vi "Status.Builder.State.New.vi"(8 "error in (no error)":errorcluster, 11 "Builder State in":refnum<class "Status.Builder.State.lvclass">) -> (0 "error out":errorcluster, 3 "Builder State out":refnum<class "Status.Builder.State.lvclass">)   [LabVIEW 2016, in "DSF.Engine.lvlib" / "Status.Builder.State.lvclass"]
uses:
  Status.Builder.State.lvclass
  C:/Git/Sourcetree/DSF/Source/Submodules/Memory/Source/Classes/Standard Types/Memory.Pointer.U8.lvclass
  Submodules/Memory/Source/Classes/Internal/Memory.Pointer.Internal.New.vi
  Submodules/Memory/Source/Classes/Internal/Memory.Pointer.Internal.New.1B.vi
  Submodules/Memory/Source/Classes/Standard Types/Memory.Pointer.U8.lvclass
  C:/Git/Sourcetree/DSF/Source/Submodules/Memory/Source/Classes/Internal/Memory.Pointer.Internal.lvclass
  Submodules/Memory/Source/Classes/Internal/Memory.Pointer.Internal.Allocate.vi
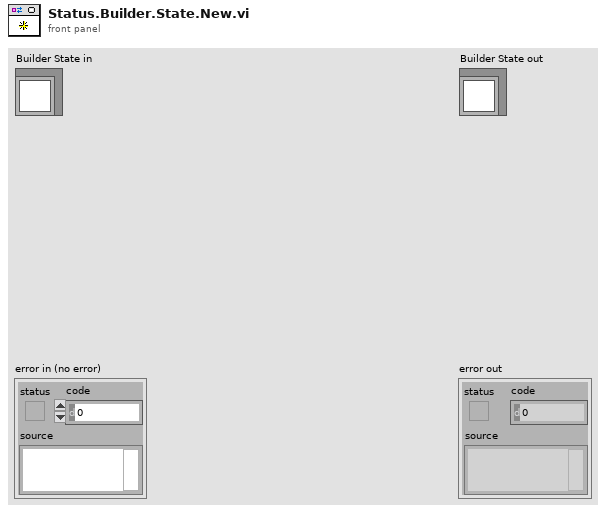
[diagram p1: front panel]
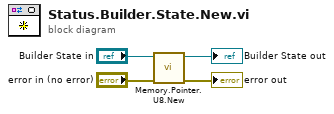
[diagram p0: block diagram]
diagram:
  n1 = call "Memory.Pointer.U8.New.vi"("error in (no error)"="error in (no error)", "U8 Pointer in"="Builder State in") -> ("error out"=→"error out":errorcluster, "U8 Pointer out"=→"Builder State out":refnum<class "Status.Builder.State.lvclass">)  [unwired: 8 in]
